vi "New No SideMenu.vi"(8 "Error In":errorcluster) -> (0 "Error Out":errorcluster, 3 "No SideMenu":refnum<class "No SideMenu.lvclass">)   [LabVIEW 2021, in "Appearance Actor.lvlib" / "No SideMenu.lvclass"]
uses:
  No SideMenu.lvclass
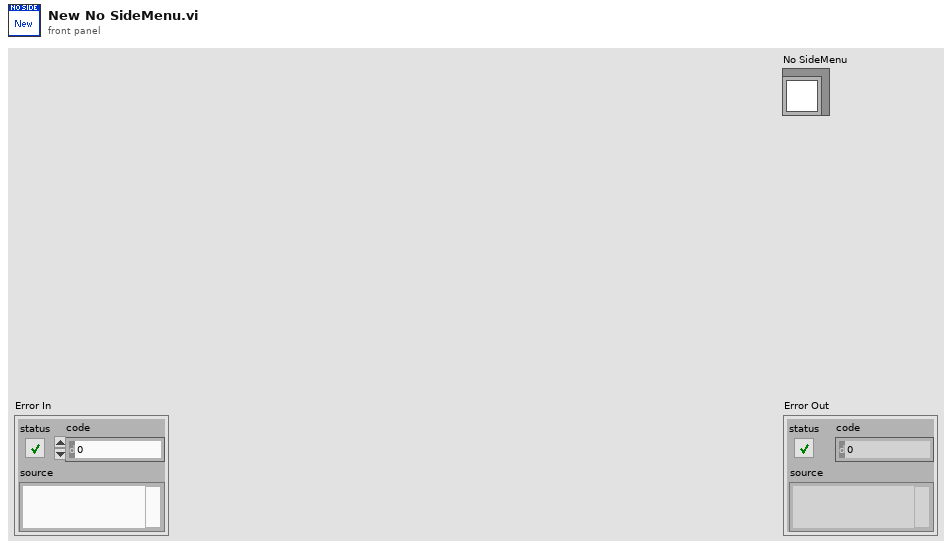
[diagram p1: front panel]
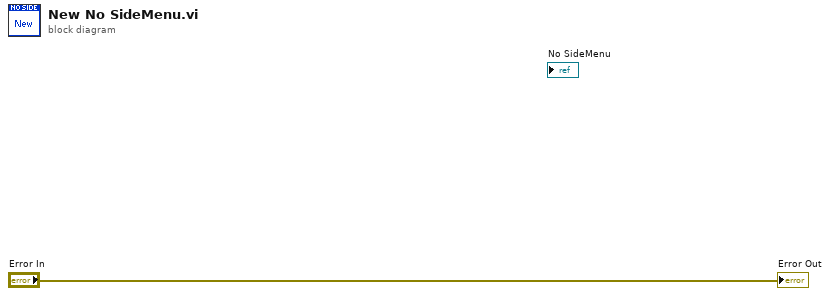
[diagram p0: block diagram]
diagram:
  "Error Out" <- "Error In"
